vi "GAIN_SELECTOR_TYPE - Type.vi"(8 "error in (no error)":errorcluster) -> (0 "error out":errorcluster, 3 "GAIN_SELECTOR_TYPE_VALUE":i32)   [LabVIEW 2015]
doc: "<b>Buffer policy settings can be only unsafe in xiAPI LabVIEW library</b>\nUNSAFE : User gets pointer to internally allocated circle buffer and data may be overwritten by device.\nSAFE : Data from device will be copied to user allocated buffer or xiApi allocated memory."
uses:
  C:/GIT/Cameras3.x/Integrations/Labview/xiLib/xiLIB_32bit/xiLIB/xiCamLib/API/x86/xiApi.NET.dll
  xiLIB_32bit/xiLIB/xiCamLib/API/x86/xiApi.NET.dll
  GAIN_SELECTOR_TYPE.ctl
panel:
  in  "GAIN_SELECTOR_TYPE":T1
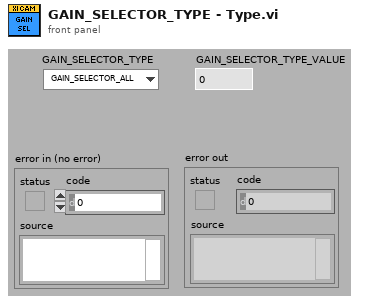
[diagram p1: front panel]
types:
  T1 = typedef "GAIN_SELECTOR_TYPE.ctl" = enum16{"GAIN_SELECTOR_ALL", "GAIN_SELECTOR_ANALOG_ALL", "GAIN_SELECTOR_DIGITAL_ALL"}
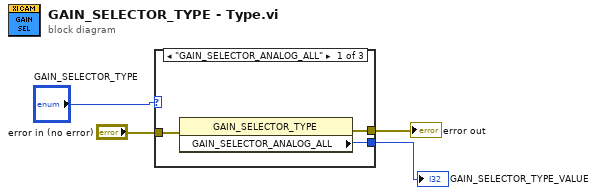
[diagram p0: block diagram]
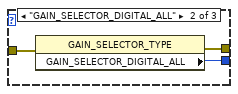
[diagram p2: hidden frame]
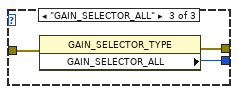
[diagram p3: hidden frame]
diagram:
  n1 = case shown="\"GAIN_SELECTOR_ANALOG_ALL\"" "GAIN_SELECTOR_TYPE" {
    tunnel: "error in (no error)" -> [w7 w10 w13]
    tunnel: [w6 w9 w12] -> w3
    tunnel: [w5 w8 w11] -> w2
    frame "GAIN_SELECTOR_ANALOG_ALL" {
      n2 = property class="GAIN_SELECTOR_TYPE"(error in=w7) -> (error out=w6:errorcluster, "GAIN_SELECTOR_ANALOG_ALL"=w5:i32)  [unwired: 1 in, 1 out]
    }
    frame "GAIN_SELECTOR_DIGITAL_ALL" {
      n3 = property class="GAIN_SELECTOR_TYPE"(error in=w10) -> (error out=w9:errorcluster, "GAIN_SELECTOR_DIGITAL_ALL"=w8:i32)  [unwired: 1 in, 1 out]
    }
    frame "GAIN_SELECTOR_ALL" {
      n4 = property class="GAIN_SELECTOR_TYPE"(error in=w13) -> (error out=w12:errorcluster, "GAIN_SELECTOR_ALL"=w11:i32)  [unwired: 1 in, 1 out]
    }
  }
  "error out" <- w3
  "GAIN_SELECTOR_TYPE_VALUE" <- w2
